vi "ValidateExp.vi"(8 "error in (no error)":errorcluster, 11 "Interface in":refnum<class "Interface.lvclass">) -> (0 "error out":errorcluster, 3 "Interface out":refnum<class "Interface.lvclass">)   [LabVIEW 2018, in "Interface.lvclass"]
uses:
  Interface.lvclass
  Interface.lvclass/Interface.ctl
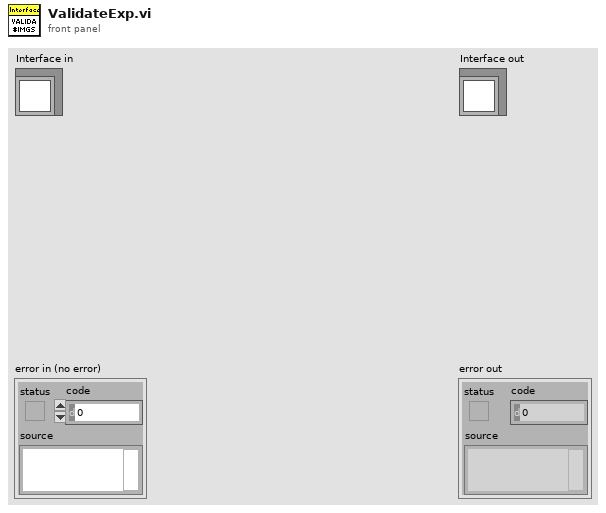
[diagram p1: front panel]
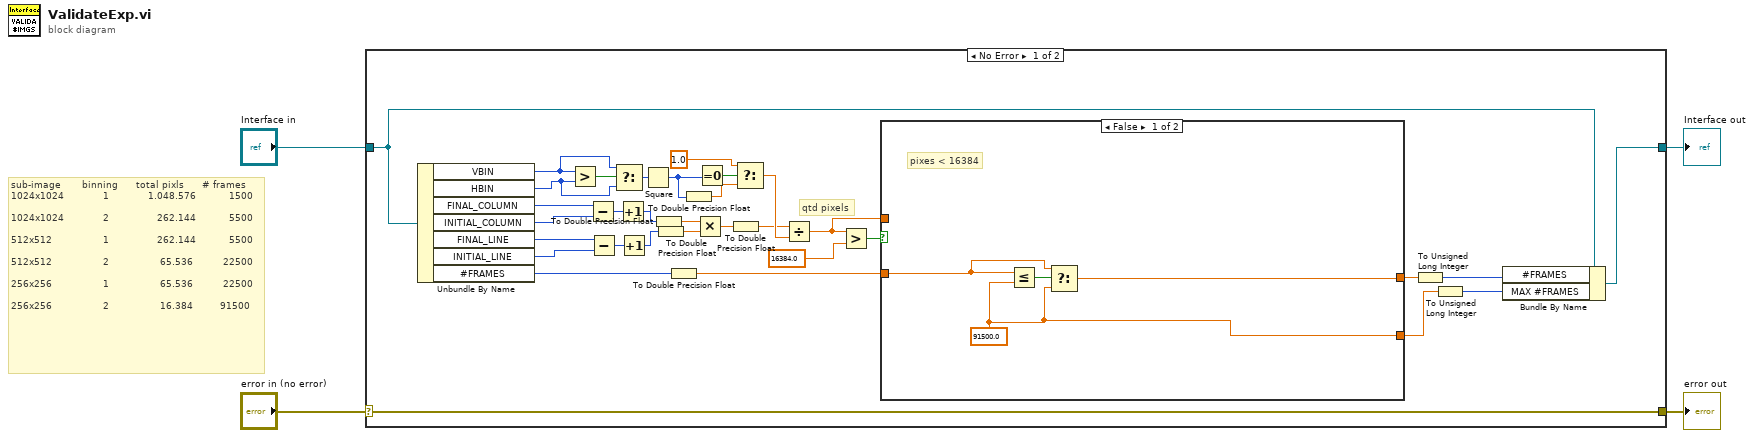
[diagram p0: block diagram]
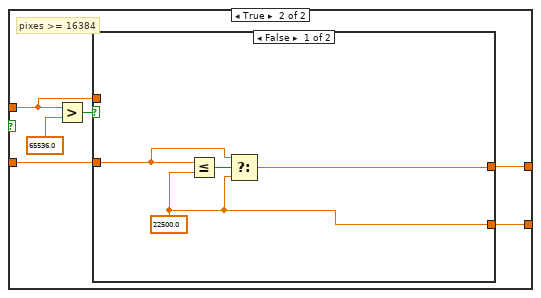
[diagram p2: hidden frame]
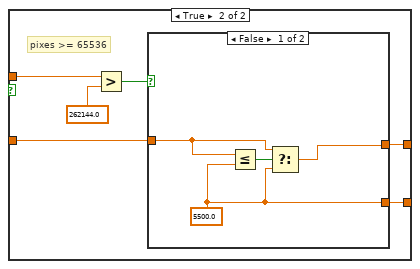
[diagram p3: hidden frame]
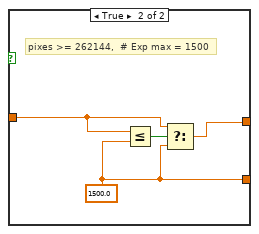
[diagram p4: hidden frame]
diagram:
  # "sub-image       binning      total pixls      # frames\n1024x1024             1             1.048.576           1500\n\n1024x1024             2                262.144           5500\n\n512x512                 1                262.144           5500\n\n512x512                 2                 65.536          22500\n\n256x256                 1                 65.536          22500\n\n256x256                 2                 16.384         91500"
  n1 = case shown="No Error" "error in (no error)" {
    selector: "error in (no error)" -> [w37 w67]
    tunnel: [w37 w67] -> w3
    tunnel: [w11 w66] -> w1
    tunnel: "Interface in" -> [w13 w66]
    frame No Error {
      # "qtd pixels"
      n2 = Unbundle By Name(w13) -> ("VBIN"=w35:u16, "HBIN"=w34:u16, "FINAL_COLUMN"=w32:u16, "INITIAL_COLUMN"=w31:u16, "FINAL_LINE"=w28:u16, "INITIAL_LINE"=w27:u16, "#FRAMES"=w17:u32)
      n3 = Greater?(x=w35, y=w34) -> (0:w36:bool)
      n4 = Subtract(x=w32, y=w31) -> (x-y=w30:u16)
      n5 = Subtract(x=w28, y=w27) -> (x-y=w29:u16)
      n6 = Select(t=w35, s=w36, f=w34) -> (s? t:f=w33:u16)
      n7 = Increment(x=w30) -> (x+1=w26:u16)
      n8 = Increment(x=w29) -> (x+1=w25:u16)
      n9 = Square(x=w33) -> (x^2=w21:u16)
      n10 = To Double Precision Float(number=w26) -> (double precision float=w8:dbl)
      n11 = To Double Precision Float(number=w25) -> (double precision float=w7:dbl)
      n12 = To Double Precision Float(number=w17) -> (double precision float=w16:dbl)
      n13 = To Double Precision Float(number=w21) -> (double precision float=w15:dbl)
      n14 = Multiply(x=w8, y=w7) -> (x*y=w24:dbl)
      n15 = Equal To 0?(x=w21) -> (x = 0?=w23:bool)
      n16 = To Double Precision Float(number=w24) -> (double precision float=w14:dbl)
      n17 = Select(t=1.0, s=w23, f=w15) -> (s? t:f=w20:dbl)
      n18 = Divide(x=w14, y=w20) -> (x/y=w9:dbl)
      n19 = Greater?(x=w9, y=16384.0) -> (0:w18:bool)
      n20 = case shown="False" w18 {
        tunnel: w16 -> [w40 w45]
        tunnel: [w39 w44] -> w12
        tunnel: w9 -> [_ w43]
        tunnel: [w38 w42] -> w6
        frame False {
          w38 = 91500.0
          # "pixes < 16384"
          n21 = Less Or Equal?(x=w40, y=w38) -> (x <= y?=w41:bool)
          n22 = Select(t=w40, s=w41, f=w38) -> (s? t:f=w39:dbl)
        }
        frame True {
          # "pixes >= 16384"
          n23 = Greater?(x=w43, y=65536.0) -> (0:w46:bool)
          n24 = case shown="False" w46 {
            tunnel: w45 -> [w50 w54]
            tunnel: [w49 w53] -> w44
            tunnel: w43 -> [_ w56]
            tunnel: [w48 w52] -> w42
            frame False {
              w48 = 22500.0
              n25 = Less Or Equal?(x=w50, y=w48) -> (x <= y?=w51:bool)
              n26 = Select(t=w50, s=w51, f=w48) -> (s? t:f=w49:dbl)
            }
            frame True {
              # "pixes >= 65536"
              n27 = Greater?(x=w56, y=262144.0) -> (0:w55:bool)
              n28 = case shown="False" w55 {
                tunnel: w54 -> [w60 w64]
                tunnel: [w59 w63] -> w53
                tunnel: [w58 w62] -> w52
                frame False {
                  w58 = 5500.0
                  n29 = Less Or Equal?(x=w60, y=w58) -> (x <= y?=w61:bool)
                  n30 = Select(t=w60, s=w61, f=w58) -> (s? t:f=w59:dbl)
                }
                frame True {
                  w62 = 1500.0
                  # "pixes >= 262144,  # Exp max = 1500"
                  n31 = Less Or Equal?(x=w64, y=w62) -> (x <= y?=w65:bool)
                  n32 = Select(t=w64, s=w65, f=w62) -> (s? t:f=w63:dbl)
                }
              }
            }
          }
        }
      }
      n33 = To Unsigned Long Integer(number=w12) -> (unsigned 32bit integer=w10:u32)
      n34 = To Unsigned Long Integer(number=w6) -> (unsigned 32bit integer=w5:u32)
      n35 = Bundle By Name(cluster=w13, "#FRAMES"=w10, "MAX #FRAMES"=w5) -> (w11:refnum<class "Interface.lvclass">)
    }
    frame Error {
    }
  }
  "error out" <- w3
  "Interface out" <- w1
